vi "MergeStrings.vi"() -> ()   [LabVIEW 2014]
panel:
  out "String 5":string
  out "String 4":string
  out "String 3":string
  in  "String 2":string
  in  "String 1":string
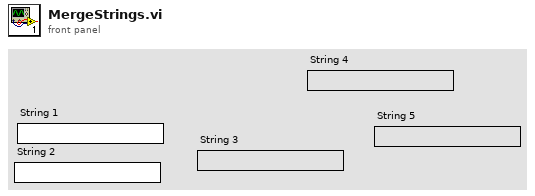
[diagram p1: front panel]
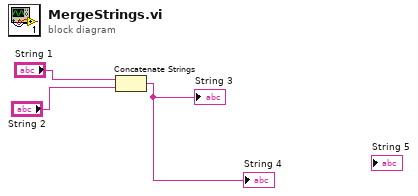
[diagram p0: block diagram]
diagram:
  n1 = Concatenate Strings("String 1", "String 2") -> (→"String 3" →"String 4":string)
